vi "Test Copy Image Greyscale Mask Greyscale.vi"(8 "error in (no error)":errorcluster, 11 "Test Case In":refnum<class "01_Image.lvclass">) -> (0 "error out":errorcluster, 3 "Test Case Out":refnum<class "01_Image.lvclass">)   [LabVIEW 2020, in "test.lvlib" / "01_Image.lvclass"]
uses:
  01_Image.lvclass
  C:/Program Files (x86)/National Instruments/LabVIEW 2026/vi.lib/Astemes/LUnit/Test Case.lvclass
  common/Image Size (Integer).ctl
  <vilib>/Astemes/LUnit/Test Case.lvclass/Test Case.ctl
  image/New Image (Greyscale Preallocated).vi
  image/Copy Array to Image (Greyscale).vi
  image/Copy Image (Greyscale with Mask).vi
  4993e8ee-a06a-463a-9684-69129f64d5ce.vi
  image/New Image (Greyscale Preallocated).vi/6598b9e0-8a08-46f5-91fd-ca1b87217137.vi
  image/Copy Image (Greyscale with Mask).vi/1519c485-f8d8-4564-b4f6-4c035770646f.vi
  <vilib>/Astemes/LUnit/Core/LUnit Test Case/Private/Append Pass Result.vi
  <vilib>/Astemes/LUnit/Core/LUnit Test Case/Private/Append Fail Result.vi
  4993e8ee-a06a-463a-9684-69129f64d5ce.vi/9c5d11cd-9439-4240-a1ee-d9baace9c924.vi
  <vilib>/Astemes/LUnit/Core/LUnit Test Case/Private/Run In UI.vi
  <vilib>/Utility/error.llb/Clear Errors.vi
  <vilib>/Utility/error.llb/Error Cluster From Error Code.vi
  <vilib>/picture/pixmap.llb/Flatten Pixmap.vi
  image/image.lvlib
  common/common.lvlib
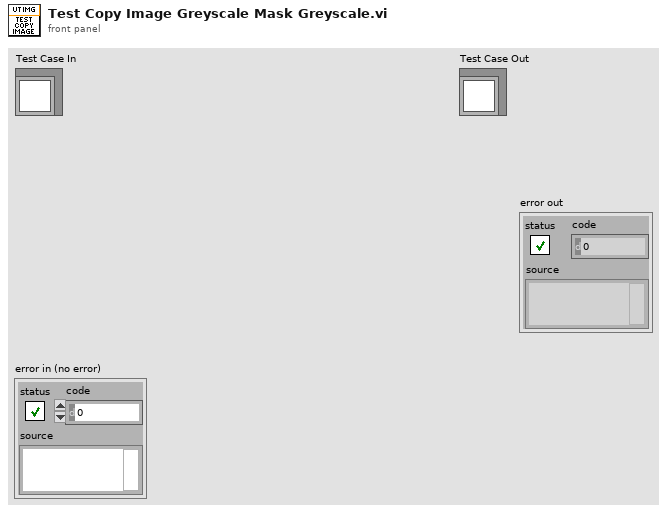
[diagram p1: front panel]
types:
  T1 = typedef "common.lvlib/Image Size (Integer).ctl" = cluster{"Width":u16, "Height":u16}
  T2 = typedef "image.lvlib/Greyscale Image.ctl" = refnum<data-value>
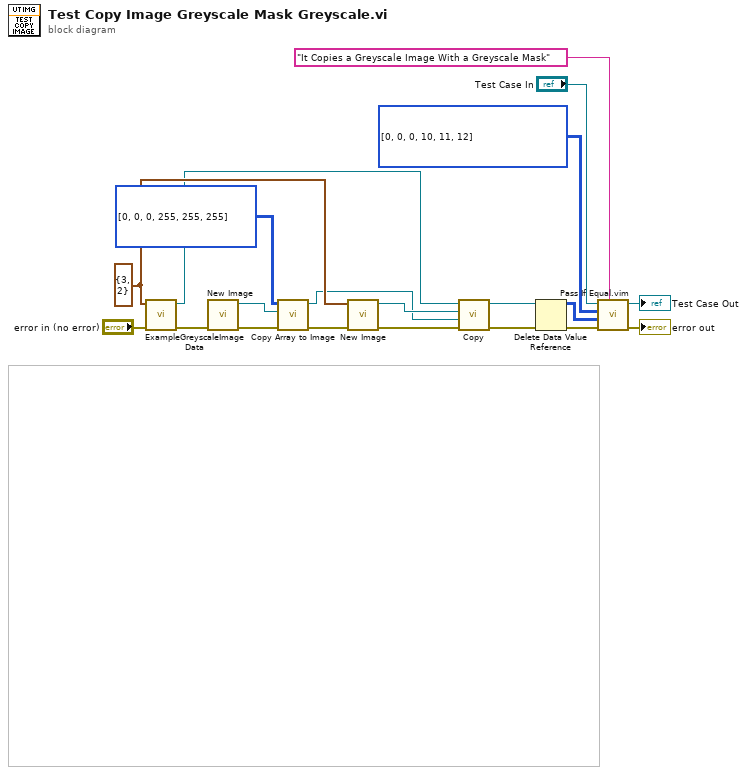
[diagram p0: block diagram]
diagram:
  w12 = T1 {"Width"=3, "Height"=2} ("Preallocated Image Size (Default - 0,0)")
  n1 = call "ExampleGreyscaleImageData.vi"("error in (no error)"="error in (no error)", "Image Size"=w12) -> ("error out"=w10:errorcluster, "Greyscale Destination Image"=w3:T2)  [unwired: 6 in, 2 out]
  n2 = call-poly "New Image.vi"("error in (no error)"=w10) -> ("error out"=w15:errorcluster, "Greyscale Image"=w8:T2)  [unwired: 9 in]
  n3 = call-poly "Copy Array to Image.vi"("error in (no error)"=w15, "Greyscale Destination Image in"=w8, "U8 Greyscale Data"=u8[][] [[0, 0, 0], [255, 255, 255]] ("Source")) -> ("error out"=w9:errorcluster, "Greyscale Destination Image"=w5:T2)  [unwired: 7 in]
  n4 = call-poly "New Image.vi"("error in (no error)"=w9, "Preallocated Image Size (Default 0,0)"=w12) -> ("error out"=w4:errorcluster, "Greyscale Image"=w6:T2)  [unwired: 8 in]
  n5 = call-poly "Copy.vi"("error in (no error)"=w4, "Greyscale Image Mask in"=w5, "Greyscale Image Destination in"=w6, "Greyscale Image Source in"=w3) -> ("error out"=w16:errorcluster, "Greyscale Image Destination"=w14:T2)  [unwired: 6 in]
  n6 = Delete Data Value Reference(data value reference=w14, error in=w16) -> (data value=w1:u8[][], error out=w13:errorcluster)
  n7 = call "Pass If Equal.vim"("Description"="It Copies a Greyscale Image With a Greyscale Mask", "error in (no error)"=w13, "Actual"=w1, "Expected"=u8[][] [[0, 0, 0], [10, 11, 12]] ("data value"), "LUnit Test Case In"="Test Case In") -> ("error out"=→"error out":errorcluster, "LUnit Test Case Out"=→"Test Case Out":refnum<class "01_Image.lvclass">)  [unwired: 5 in]
